vi "Change_button_color.vi"(5 "Button":refnum<vi>, 9 "Text":string, 11 "Colors [4]":cluster{"Color Box":u32, "Color Box":u32}[](array[cluster])=[{"Color Box"=15203839, "Color Box"=16119285}, {"Color Box"=16777215, "Color Box"=16777215}, {"Color Box"=0, "Color Box"=0}, {"Color Box"=65511, "Color Box"=16770137}]) -> ()   [LabVIEW 2023]
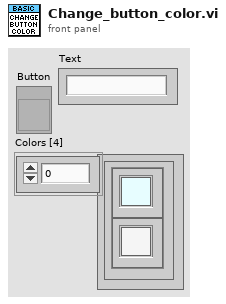
[diagram p1: front panel]
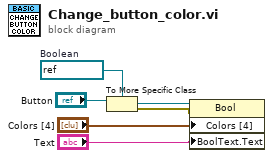
[diagram p0: block diagram]
diagram:
  w6 = refnum<vi> refnum  # Boolean
  n1 = To More Specific Class(target class=w6, reference="Button") -> (specific class reference=w4:refnum<vi>, error out=w3:errorcluster)  [unwired: 1 in]
  n2 = property class="Bool"(reference=w4, error in=w3, "Colors [4]"="Colors [4]", "BoolText.Text"="Text") -> ()  [unwired: 2 out]
